vi "WPI_JoystickTankMapping.vi"(6 "Max Output":dbl, 7 "Square Inputs":bool, 9 "Right axis value":dbl, 10 "Left axis value":dbl) -> (1 "Right Motor Value":dbl, 2 "Left Motor Value":dbl)   [LabVIEW 2017]
doc: "Maps joysticks for tank driving. It uses the y-axis values of two joysticks. Each specifies the power to apply to the motors one side of the robot."
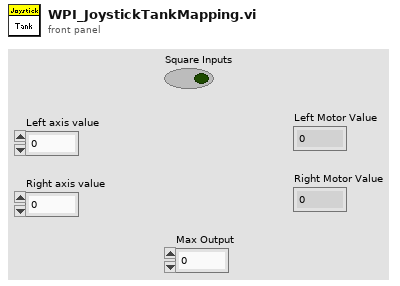
[diagram p1: front panel]
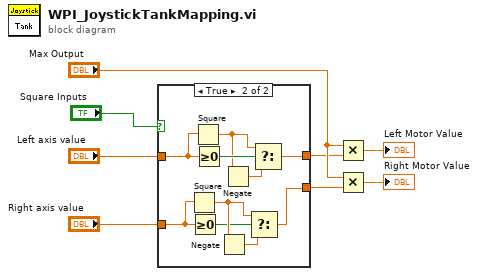
[diagram p0: block diagram]
diagram:
  n1 = case shown="True" "Square Inputs" {
    tunnel: "Left axis value" -> [w10 w20]
    tunnel: [w10 w16] -> w2
    tunnel: [w9 w12] -> w6
    tunnel: "Right axis value" -> [w9 w11]
    frame False {
    }
    frame True {
      n2 = Square(x=w11) -> (x^2=w14:dbl)
      n3 = Greater Or Equal To 0?(x=w11) -> (x >= 0?=w13:bool)
      n4 = Square(x=w20) -> (x^2=w18:dbl)
      n5 = Greater Or Equal To 0?(x=w20) -> (x >= 0?=w19:bool)
      n6 = Negate(x=w14) -> (-x=w15:dbl)
      n7 = Negate(x=w18) -> (-x=w17:dbl)
      n8 = Select(t=w14, s=w13, f=w15) -> (s? t:f=w12:dbl)
      n9 = Select(t=w18, s=w19, f=w17) -> (s? t:f=w16:dbl)
    }
  }
  n10 = Multiply(x="Max Output", y=w2) -> (x*y=→"Left Motor Value":dbl)
  n11 = Multiply(x="Max Output", y=w6) -> (x*y=→"Right Motor Value":dbl)
